vi "Data Notifier.vi"(7 "State":T1=enum."Get", 8 "error in":errorcluster, 11 "MAP DVR":refnum<data-value>) -> (0 "error out":errorcluster, 3 "Data Map":variant)   [LabVIEW 2014, in "Controller.lvlib" / "Controller.lvclass"]
doc: "This VI facillitates communication between the web services and the controller. This VI stores a notifier that is used to ship data from the controller to the web services."
uses:
  Controller.lvclass
  Controls/Notifier Enum.ctl
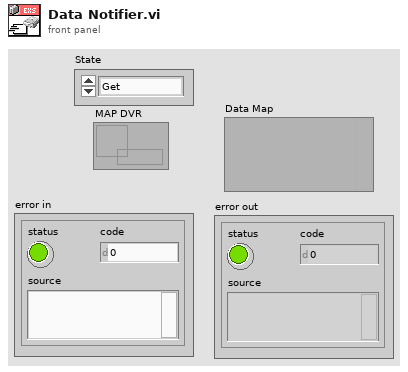
[diagram p1: front panel]
types:
  T1 = typedef "Notifier Enum.ctl" = enum16{"Initialize", "Get", "Set", "Close"}
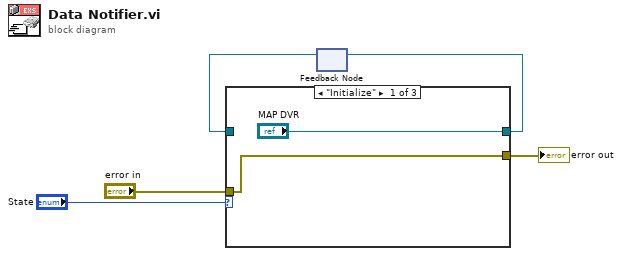
[diagram p0: block diagram]
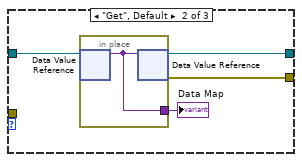
[diagram p2: hidden frame]
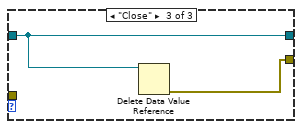
[diagram p3: hidden frame]
diagram:
  n1 = feedback #1() -> (w4:refnum<data-value>)  [unwired: 1 in]
  n2 = case shown="\"Initialize\"" "State" {
    tunnel: ["MAP DVR" w10 w14] -> w5
    tunnel: w4 -> [_ w11 w14]
    tunnel: [w6 w9 w13] -> w3
    tunnel: "error in" -> [w6 _ _]
    frame "Initialize" {
    }
    frame "Get", Default {
      n3 = in-place {
        in-place-border: [w12] -> w8
        n4 = in-place-dvr #2(w11) -> (w12:variant)  [unwired: 1 out]
        n5 = in-place-dvr #2(w12) -> (w10:refnum<data-value>, w9:errorcluster)
      }
      "Data Map" <- w8
    }
    frame "Close" {
      n6 = Delete Data Value Reference(data value reference=w14) -> (error out=w13:errorcluster)  [unwired: 1 in, 1 out]
    }
  }
  "error out" <- w3
  n7 = feedback-in #1(w5) -> ()
